vi "Pins Names Write.vi"(4 "error in (no error)":errorcluster, 5 "Value":string[](array[string]), 6 "Container State":T2, 7 "Display State In":T1) -> (0 "error out":errorcluster, 3 "Display State Out":T1)   [LabVIEW 2021, in "myRIO MXP.xctl"]
uses:
  <vilib>/myRIO/Common/Instrument Driver Framework/Utilities/xctls/myRIO MXP/myRIO MXP.xctl
  <vilib>/_xctls/Container State.ctl
  <vilib>/myRIO/Common/Instrument Driver Framework/Utilities/xctls/myRIO MXP/State.ctl
  <vilib>/myRIO/Common/Instrument Driver Framework/Utilities/xctls/utilities/vis/myRIOXC Error Strings Global.vi
  <vilib>/_xctls/XControlSupport.lvlib
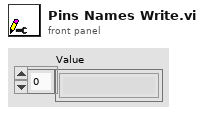
[diagram p1: front panel]
types:
  T1 = typedef "myRIO MXP.xctl/State.ctl" = cluster{"Pin Disabled?":enum8{"Enabled", "Disabled", "Disabled and Grayed Out"}[], "Pin Name":string[]}
  T2 = typedef "XControlSupport.lvlib/Container State.ctl" = cluster{"Indicator?":bool, "Run Mode?":bool, " Refnum":refnum<vi>}
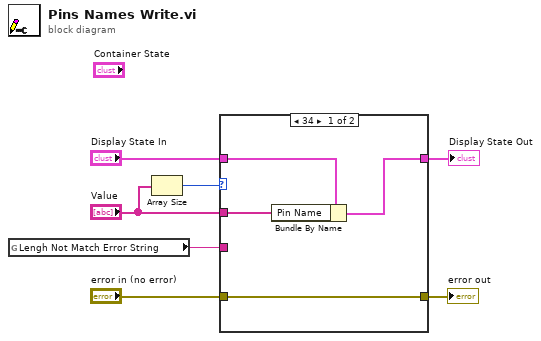
[diagram p0: block diagram]
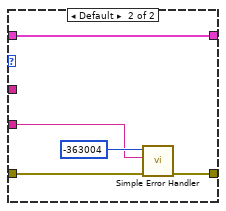
[diagram p2: hidden frame]
diagram:
  n1 = global read "myRIOXC Error Strings Global.vi" "Lengh Not Match Error String"() -> (w1:string)
  n2 = Array Size(array="Value") -> (size(s)=w6:i32)
  n3 = case shown="34" w6 {
    tunnel: "Display State In" -> [w11 w16]
    tunnel: [w10 w16] -> w5
    tunnel: "Value" -> [w9 _]
    tunnel: "error in (no error)" -> [w8 w14]
    tunnel: [w8 w13] -> w2
    tunnel: w1 -> [_ w12]
    frame 34 {
      n4 = Bundle By Name(cluster=w11, "Pin Name"=w9) -> (w10:T1)
    }
    frame Default {
      n5 = call <vilib>:"Simple Error Handler.vi"("error code (no error:0)"=-363004, "error source (\" \")"=w12, "error in (no error)"=w14) -> ("error out"=w13:errorcluster)  [unwired: 2 in, 4 out]
    }
  }
  "error out" <- w2
  "Display State Out" <- w5
